vi "Reset by IC10.vi"(8 "error in":errorcluster) -> (0 "error out":errorcluster, 1 "VRESET Pass/Fail":bool, 2 "VNORESET Pass/Fail":bool, 3 "Pass/Fail":bool)   [LabVIEW 2009]
uses:
  Digit IO PCI 6503/Digit IO control.ctl
  Global/Global 1.vi
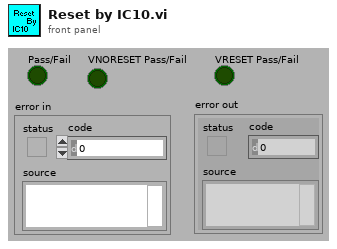
[diagram p1: front panel]
types:
  T1 = typedef "Digit IO control.ctl" = enum16{"Pull X1_4 Low", "Disconnect Pull X1_4 Low", "Down Cylinder", "Disconnect Down Cylinder", "Load X1_1_5", "Disconnect Load X1_1_5", "Measu X1_1_5", "Disconnect Measu X1_1_5", "Measu Z1_1_5", "Disconnect Measu Z1_1_5", "Power X1_1", "Disconnect Power X1_1", "RS232 Power", "Disconnect RS232 Power", "Card Cylinder", "Disconnect Card Cylinder", "Fail LED", "Disconnect Fail LED", "LCA Power", "Disconnect LCA Power", "BeyondCylinderDowndigit", "Disconnect BeyondCylinderDowendigit", "Frequency", "Disconnect Frequency", "Measu Current", "Disconnect Measu Current", "Measu current_1", "Disconnect Measu current_1", "Digit ALL", "Disconnect Digit ALL", "PASS LED", "Disconnect PASS LED", "Load Z1_1_3", "Disconnect Load Z1_1_3", "RS232 Connect", "Disconnect RS232 Connect", "Power Z1_7", "Disconnect Power Z1_7", "Pull Z_1_5  low", "Disconnect Pull Z_1_5  low", "Connect LCA_1", "Disconnect LCA_1", "short LCA", "Disconnect short LCA", "PT100", "Disconnect PT100", "NO connect", "Disconnect NO connect"}
  T2 = cluster{"People":string, "product  number":string, "Test time":string, "VHeatFuse_noload":string, "VHeatFuse_load":string, "VoverrideDiode":string, "Test firmware upload via X1":string, "TemperAddress":string, "Troom":string, "TLCU":string, "Adjustment factor":string, "MeasuredFreq":string, "I2C communication":string, "Light-emitting diode on Z2":string, "Battery warning/inhibit":string, "Reset by IC10":string, "External EEPROM":string, "RFID card detection and reading RFID":string, "Production parameters in internal EEPROM":string, "Current consumption in sleep mode":string, "Application and database upload":string, "Test result":string, "Table head[22]":string, "Table head[23]":string}
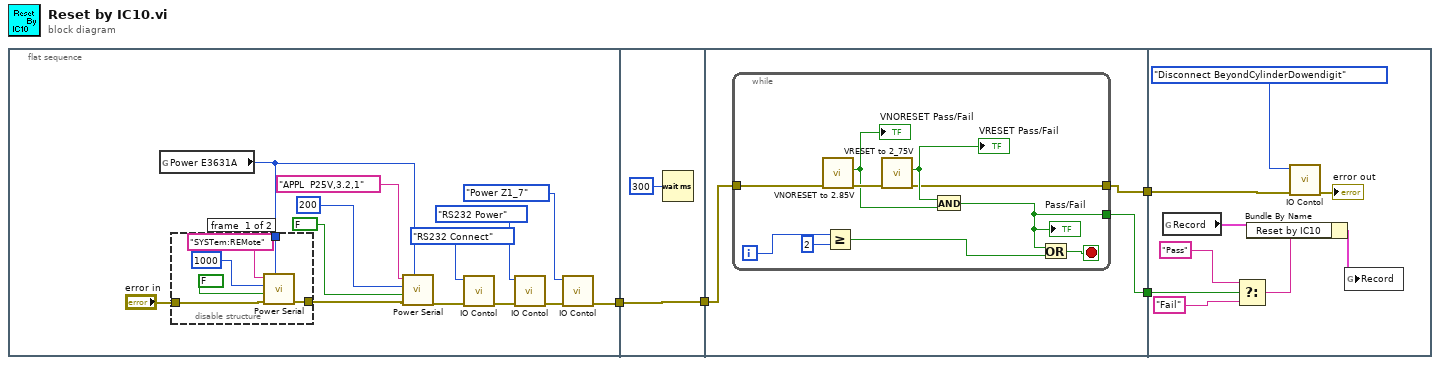
[diagram p0: block diagram]
diagram:
  n1 = flat-sequence {
    tunnel: [w8] -> w1
    tunnel: w1 -> [w26]
    tunnel: [w26] -> w3
    tunnel: w3 -> [w29]
    tunnel: [w28] -> w4
    tunnel: [w27] -> w2
    tunnel: w4 -> [w40]
    tunnel: w2 -> [w43]
    frame #0 {
      n2 = global read "Global 1.vi" "Power E3631A"() -> (w15:i32)
      n3 = disable-structure shown="Enabled" {
        disable-tunnel: w15 -> [w23 _]
        disable-tunnel: "error in" -> [w19 w24]
        disable-tunnel: [w18 w24] -> w9
        frame #0 {
          n4 = call "Power Serial.vi"("VISA Resource Address"=w23, "error in (no error)"=w19, "Rd?"=FALSE, "Delay"=1000, "IN"="SYSTem:REMote" ("In")) -> ("error out"=w18:errorcluster)  [unwired: 5 in, 1 out]
        }
        frame #1 {
        }
      }
      n5 = call "Power Serial.vi"("VISA Resource Address"=w15, "error in (no error)"=w9, "Rd?"=FALSE, "Delay"=200, "IN"="APPL  P25V,3.2,1" ("In")) -> ("error out"=w17:errorcluster)  [unwired: 6 out]
      n6 = call "IO Contol.vi"("error in"=w17, "IO Operation"=Digit_IO_control."RS232 Connect" ("Enum")) -> ("error out"=w16:errorcluster)  [unwired: 9 out]
      n7 = call "IO Contol.vi"("error in"=w16, "IO Operation"=Digit_IO_control."RS232 Power" ("Enum")) -> ("error out"=w14:errorcluster)  [unwired: 9 out]
      n8 = call "IO Contol.vi"("error in"=w14, "IO Operation"=Digit_IO_control."Power Z1_7" ("Enum")) -> ("error out"=w8:errorcluster)  [unwired: 9 out]
    }
    frame #1 {
      n9 = Wait (ms)(milliseconds to wait=u32 300) -> ()  [unwired: 1 out]
    }
    frame #2 {
      n10 = while {
        tunnel: w29 -> [w39]
        tunnel: [w31] -> w28
        tunnel: [w30] -> w27
        i -> [w37]
        stop <- w35 stop-if-true
        n11 = call "VNORESET to 2.85V.vi"("error in"=w39) -> ("error out"=w38:errorcluster, "Pass/Fail"=w33:bool)  [unwired: 1 in, 8 out]
        "VNORESET Pass/Fail" <- w33
        n12 = Greater Or Equal?(x=w37, y=2) -> (x >= y?=w32:bool)
        n13 = call "VRESET to 2_75V.vi"("error in"=w38) -> ("error out"=w31:errorcluster, "Pass/Fail"=w34:bool)  [unwired: 1 in, 8 out]
        "VRESET Pass/Fail" <- w34
        n14 = And(x=w34, y=w33) -> (x .and. y?=w30:bool)
        "Pass/Fail" <- w30
        n15 = Or(x=w30, y=w32) -> (x .or. y?=w35:bool)
      }
    }
    frame #3 {
      n16 = global read "Global 1.vi" "Record"() -> (w46:T2)
      n17 = Select(t="Pass", s=w43, f="Fail") -> (s? t:f=w42:string)
      n18 = Bundle By Name(cluster=w46, "Reset by IC10"=w42) -> (w41:T2)
      n19 = call "IO Contol.vi"("error in"=w40, "IO Operation"=Digit_IO_control."Disconnect BeyondCylinderDowendigit" ("Enum")) -> ("error out"=→"error out":errorcluster)  [unwired: 9 out]
      n20 = global write "Global 1.vi" "Record"(w41) -> ()
    }
  }
